vi "kD2ASingleVal.vi"(8 "DIO Port Selection":T1, 11 "Single Input Element":u16) -> ()   [LabVIEW 2018, in "kevLib2010.lvlib"]
uses:
  kevLib2010.lvlib
  <vilib>/eio/EIONode/EIONode.xnode
  <vilib>/rvi/eio/common/nirviEmuTemplateMethod_errors.vi
  KD2A Port Sel.ctl
panel:
  # "Note this input MUST Follow A specific Format\n[ Loc[4] Val[12] ] \nwhere Val is shifted"
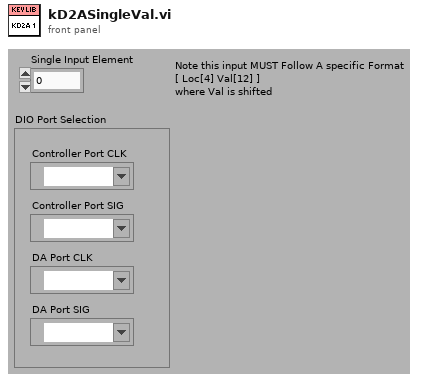
[diagram p1: front panel]
types:
  T1 = typedef "kevLib2010.lvlib/KD2A Port Sel.ctl" = cluster{"Controller Port CLK":refnum<k21>, "Controller Port SIG":refnum<k21>, "DA Port CLK":refnum<k21>, "DA Port SIG":refnum<k21>}
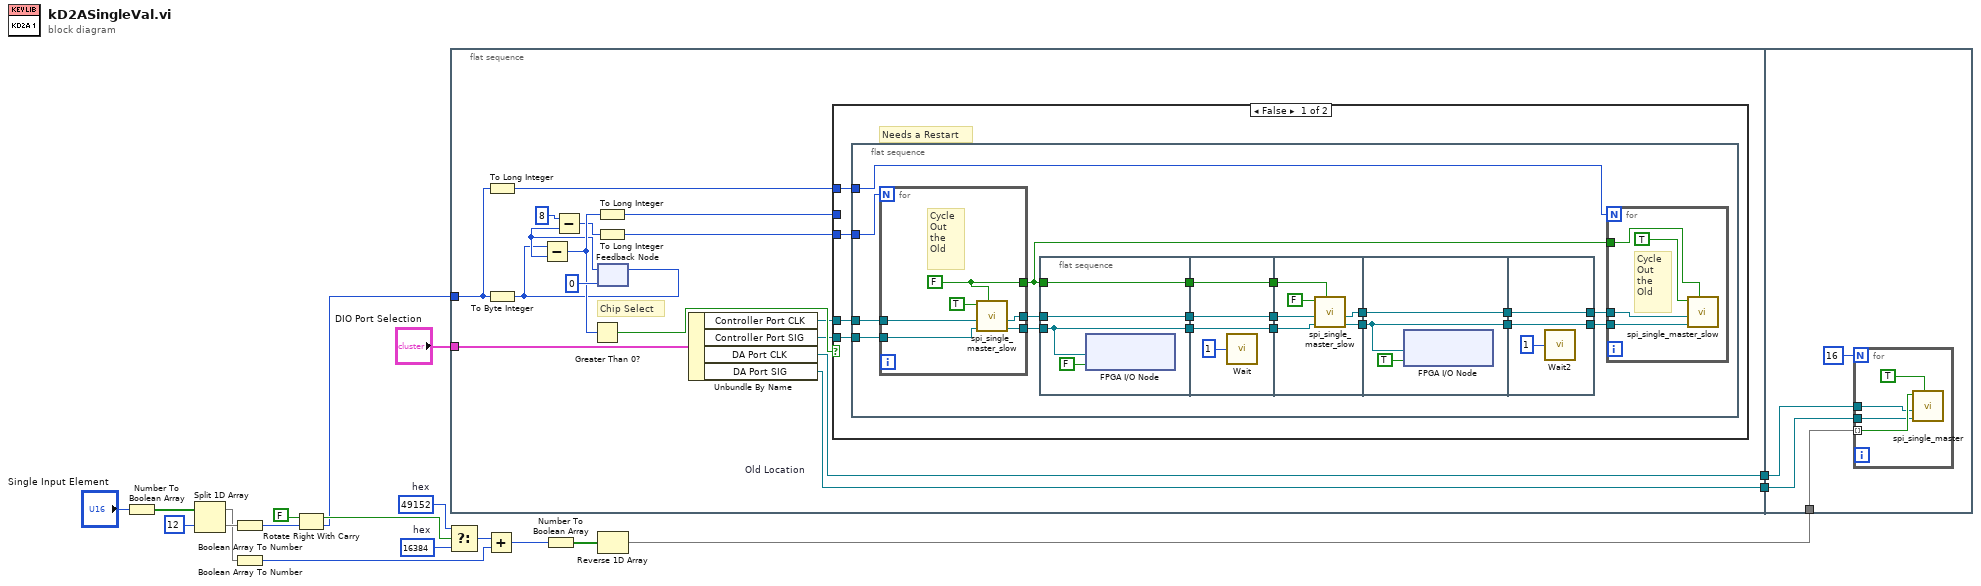
[diagram p0: block diagram]
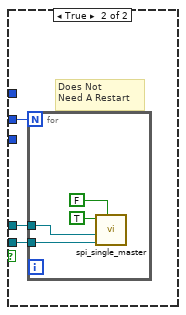
[diagram p2: hidden frame]
diagram:
  w10 = u16 49152  # hex
  w11 = u16 16384  # hex
  n1 = Number To Boolean Array(number="Single Input Element") -> (Boolean array=w4:bool[])
  n2 = Split 1D Array(array=w4, index=12) -> (first subarray=w1:bool[], second subarray=w2:bool[])
  n3 = Boolean Array To Number(Boolean array=w2) -> (number=w9:u8)
  n4 = Boolean Array To Number(Boolean array=w1) -> (number=w12:u16)
  n5 = Rotate Right With Carry(2:w9, 3:FALSE ("carry")) -> (0:w7:u8, 1:w8:bool)
  n6 = Select(t=w10, s=w8, f=w11) -> (s? t:f=w13:u16)
  n7 = flat-sequence {
    tunnel: w7 -> [w23]
    tunnel: [w22] -> w19
    tunnel: [w21] -> w18
    tunnel: "DIO Port Selection" -> [w20]
    tunnel: w16 -> [w98]
    tunnel: w19 -> [w97]
    tunnel: w18 -> [w96]
    frame #0 {
      # "Chip Select"
      n8 = To Long Integer(number=w23) -> (32bit integer=w25:i32)
      n9 = To Byte Integer(number=w23) -> (8bit integer=w24:i8)
      n10 = feedback #1 "Old Location"(i8 0) -> (w29:i8)
      n11 = Subtract(x=w24, y=w29) -> (x-y=w31:i8)
      n12 = Subtract(x=i8 8, y=w29) -> (x-y=w27:i8)
      n13 = Greater Than 0?(x=w31) -> (x > 0?=w34:bool)
      n14 = To Long Integer(number=w31) -> (32bit integer=w30:i32)
      n15 = To Long Integer(number=w27) -> (32bit integer=w26:i32)
      n16 = feedback-in #1(w24) -> ()
      n17 = Unbundle By Name(w20) -> ("Controller Port CLK"=w33:refnum<k21>, "Controller Port SIG"=w32:refnum<k21>, "DA Port CLK"=w22:refnum<k21>, "DA Port SIG"=w21:refnum<k21>)
      n18 = case shown="False" w34 {
        tunnel: w30 -> [_ w91]
        tunnel: w33 -> [w39 w90]
        tunnel: w32 -> [w37 w89]
        tunnel: w26 -> [w38 _]
        tunnel: w25 -> [w36 _]
        frame False {
          # "Needs a Restart"
          n19 = flat-sequence {
            tunnel: w39 -> [w58]
            tunnel: w38 -> [w57]
            tunnel: w37 -> [w56]
            tunnel: w36 -> [w51]
            frame #0 {
              n20 = for {
                N: w57 -> [_]
                tunnel: w58 -> [w83]
                tunnel: w56 -> [w82]
                tunnel: [w81] -> w55
                tunnel: [w80] -> w45
                tunnel: [w79] -> w54
                w79 = FALSE ("Falling Edge?")
                # "Cycle \nOut\nthe \nOld"
                n21 = call "spi_single_master_slow.vi"("Falling Edge?"=w79, "SIG Port"=w82, "CLK Port"=w83, "Signal"=TRUE) -> ("SIG Port Out"=w80:refnum<k21>, "CLK Port Out"=w81:refnum<k21>)  [unwired: 6 in]
              }
              n22 = flat-sequence {
                tunnel: w54 -> [w61]
                tunnel: w45 -> [w60]
                tunnel: w55 -> [w62]
                tunnel: [w62] -> w44
                tunnel: [w60] -> w43
                tunnel: [w61] -> w42
                tunnel: [w66] -> w50
                tunnel: [w65] -> w49
                tunnel: [w64] -> w48
                tunnel: w44 -> [w66]
                tunnel: w43 -> [w65]
                tunnel: w42 -> [w64]
                tunnel: w50 -> [w72]
                tunnel: w49 -> [w71]
                tunnel: w48 -> [w69]
                tunnel: [w68] -> w47
                tunnel: [w67] -> w46
                tunnel: w47 -> [w75]
                tunnel: w46 -> [w74]
                tunnel: [w75] -> w41
                tunnel: [w74] -> w40
                tunnel: [w77] -> w52
                tunnel: [w78] -> w53
                tunnel: w41 -> [w78]
                tunnel: w40 -> [w77]
                frame #0 {
                  n23 = xnode "FPGA I/O Node"("I/O Item"=FALSE, "FPGA I/O In"=w60) -> ()  [unwired: 1 out]
                }
                frame #1 {
                  n24 = call "Wait"("Count(Ticks)"=u8 1) -> ()  [unwired: 1 out]
                }
                frame #2 {
                  n25 = call "spi_single_master_slow.vi"("Falling Edge?"=w69, "SIG Port"=w71, "CLK Port"=w72, "Signal"=FALSE) -> ("SIG Port Out"=w67:refnum<k21>, "CLK Port Out"=w68:refnum<k21>)  [unwired: 6 in]
                }
                frame #3 {
                  n26 = xnode "FPGA I/O Node"("I/O Item"=TRUE, "FPGA I/O In"=w74) -> ()  [unwired: 1 out]
                }
                frame #4 {
                  n27 = call "Wait2"("Count(Ticks)"=u8 1) -> ()  [unwired: 1 out]
                }
              }
              n28 = for {
                N: w51 -> [_]
                tunnel: w54 -> [w87]
                tunnel: w53 -> [w86]
                tunnel: w52 -> [w85]
                # "Cycle \nOut\nthe \nOld"
                n29 = call "spi_single_master_slow.vi"("Falling Edge?"=w87, "SIG Port"=w85, "CLK Port"=w86, "Signal"=TRUE) -> ()  [unwired: 6 in, 2 out]
              }
            }
          }
        }
        frame True {
          # "Does Not \nNeed A Restart"
          n30 = for {
            N: w91 -> [_]
            tunnel: w90 -> [w93]
            tunnel: w89 -> [w92]
            n31 = call "spi_single_master.vi"("Falling Edge?"=FALSE, "SIG Port"=w92, "CLK Port"=w93, "Signal"=TRUE) -> ()  [unwired: 6 in, 2 out]
          }
        }
      }
    }
    frame #1 {
      n32 = for {
        N: 16 -> [_]
        tunnel: w98 -> [w103] mode=indexing
        tunnel: w97 -> [w101]
        tunnel: w96 -> [w100]
        n33 = call "spi_single_master.vi"("Falling Edge?"=TRUE, "SIG Port"=w100, "CLK Port"=w101, "Signal"=w103) -> ()  [unwired: 6 in, 2 out]
      }
    }
  }
  n34 = Add(x=w13, y=w12) -> (x+y=w14:u16)
  n35 = Number To Boolean Array(number=w14) -> (Boolean array=w15:bool[])
  n36 = Reverse 1D Array(array=w15) -> (reversed array=w16:bool[])
